vi "SPI_START.vi"(10 "size(s) IN":i32) -> (1 "PFIWE":bool[](array[boolean])=[TRUE, TRUE, TRUE, TRUE], 2 "SCL":bool[](array[boolean])=[TRUE, TRUE, TRUE, FALSE], 3 "SDA":bool[](array[boolean])=[TRUE, TRUE, FALSE, FALSE], 5 "size(s)":i32)   [LabVIEW 2018]
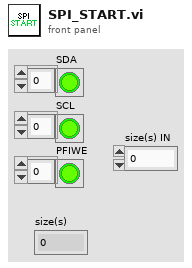
[diagram p1: front panel]
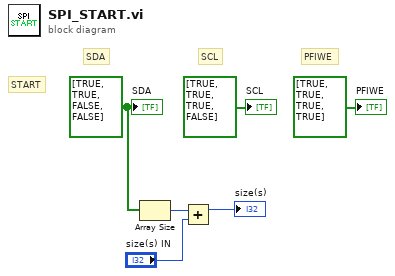
[diagram p0: block diagram]
diagram:
  w4 = bool[] [TRUE, TRUE, FALSE, FALSE]
  # "START"
  # "PFIWE"
  # "SCL"
  # "SDA"
  n1 = Array Size(array=w4) -> (size(s)=w3:i32)
  n2 = Add(x=w3, y="size(s) IN") -> (x+y=→"size(s)":i32)
  "SDA" <- w4
  "SCL" <- bool[] [TRUE, TRUE, TRUE, FALSE]
  "PFIWE" <- bool[] [TRUE, TRUE, TRUE, TRUE]
